vi "Read Deadband.vi"(8 "error in (no error)":errorcluster, 11 "Level Controller in":refnum<class "Level Controller.lvclass">) -> (0 "error out":errorcluster, 2 "Deadband":T1, 3 "Level Controller out":refnum<class "Level Controller.lvclass">)   [LabVIEW 2025, in "Level Controller.lvlib" / "Level Controller.lvclass"]
doc: "Reads the deadband range of this Level Controller."
uses:
  Level Controller.lvclass
  Deadband.ctl
  Level Controller.lvclass/Level Controller.ctl
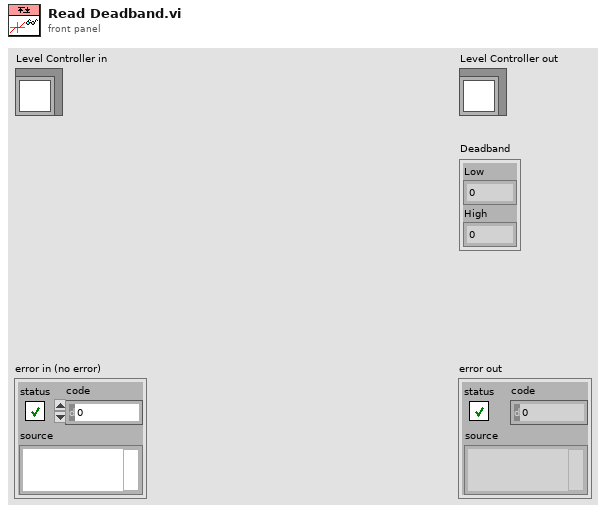
[diagram p1: front panel]
types:
  T1 = typedef "Level Controller.lvlib/Level Controller.lvclass/Deadband.ctl" = cluster{"Low":dbl, "High":dbl}
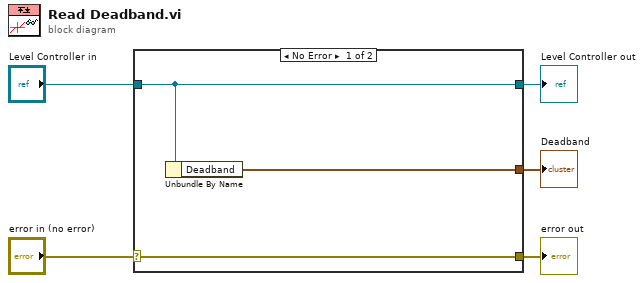
[diagram p0: block diagram]
diagram:
  n1 = case shown="No Error" "error in (no error)" {
    selector: "error in (no error)" -> [w8 w9]
    tunnel: [w8 w9] -> w4
    tunnel: [w7 w10] -> w3
    tunnel: "Level Controller in" -> [w7 w10]
    tunnel: [w6 _] -> w2
    frame No Error {
      n2 = Unbundle By Name(w7) -> ("Deadband"=w6:T1)
    }
    frame Error {
    }
  }
  "error out" <- w4
  "Level Controller out" <- w3
  "Deadband" <- w2
